vi "Update-references.vi"(6 "Control refs":refnum<vi>[](array[refnum]), 8 "error in (no error)":errorcluster, 9 "Sorted splitter references":refnum<vi>[](array[refnum]), 10 "Sorted pane references":refnum<vi>[](array[refnum]), 11 "Panes in":T1) -> (0 "error out":errorcluster, 3 "Panes out":T1)   [LabVIEW 2013, in "MaterialCharacterization.lvlib" / "MC-UI.lvclass"]
uses:
  MC-UI.lvclass
  Panes-reference.ctl
  MC-UI.lvclass/MC-UI.ctl
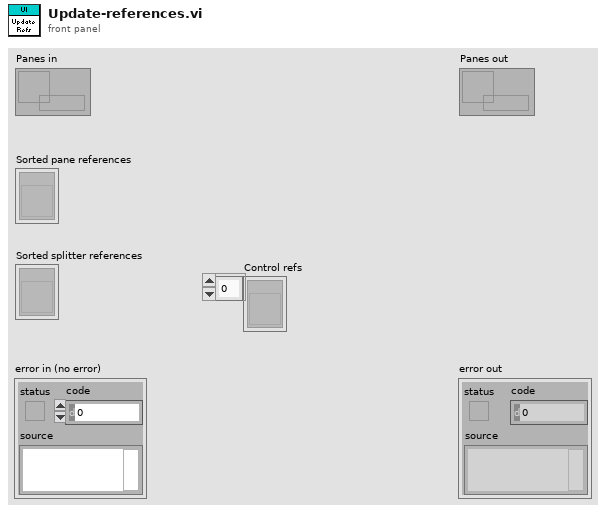
[diagram p1: front panel]
types:
  T1 = typedef "MaterialCharacterization.lvlib/MC-UI.lvclass/Panes-reference.ctl" = refnum<data-value>
  T2 = typedef "MaterialCharacterization.lvlib/HC-UI.lvclass/Pane-settings.ctl" = cluster{"Pane-name":T3, "Startup status":bool, "Current status":bool, "Splitters":T4[], "Pane-reference":refnum<vi>}
  T3 = typedef "MaterialCharacterization.lvlib/HC-UI.lvclass/Pane-names.ctl" = enum16{"Toolbar", "Help bar", "Toolbar lower border", "Center panel", "Main panel", "Settings panel", "Status bar upper border", "General state bar", "Information bar"}
  T4 = typedef "MaterialCharacterization.lvlib/HC-UI.lvclass/Splitter-settings.ctl" = cluster{"Splitter-name":T5, "Position shown":i32, "Position hidden":i32, "Splitter reference":refnum<vi>}
  T5 = typedef "MaterialCharacterization.lvlib/HC-UI.lvclass/Splitter-names.ctl" = enum16{"Upper toolbar splitter", "Help bar splitter", "Lower toolbar splitter", "Upper status bar splitter", "Lower status bar splitter", "Left status bar splitter", "Settings splitter"}
  T6 = typedef "MaterialCharacterization.lvlib/MC-UI.lvclass/Pane-settings.ctl" = cluster{"Pane-name":T7, "Startup status":bool, "Current status":bool, "Splitters":T8[], "Pane-reference":refnum<vi>}
  T7 = typedef "MaterialCharacterization.lvlib/MC-UI.lvclass/Pane-names.ctl" = enum16{"Toolbar", "Help bar", "Toolbar lower border", "Center panel", "Main panel", "Settings panel", "Status bar upper border", "General state bar", "Information bar"}
  T8 = typedef "MaterialCharacterization.lvlib/MC-UI.lvclass/Splitter-settings.ctl" = cluster{"Splitter-name":T9, "Position shown":i32, "Position hidden":i32, "Splitter reference":refnum<vi>}
  T9 = typedef "MaterialCharacterization.lvlib/MC-UI.lvclass/Splitter-names.ctl" = enum16{"Upper toolbar splitter", "Help bar splitter", "Lower toolbar splitter", "Upper status bar splitter", "Lower status bar splitter", "Left status bar splitter", "Settings splitter"}
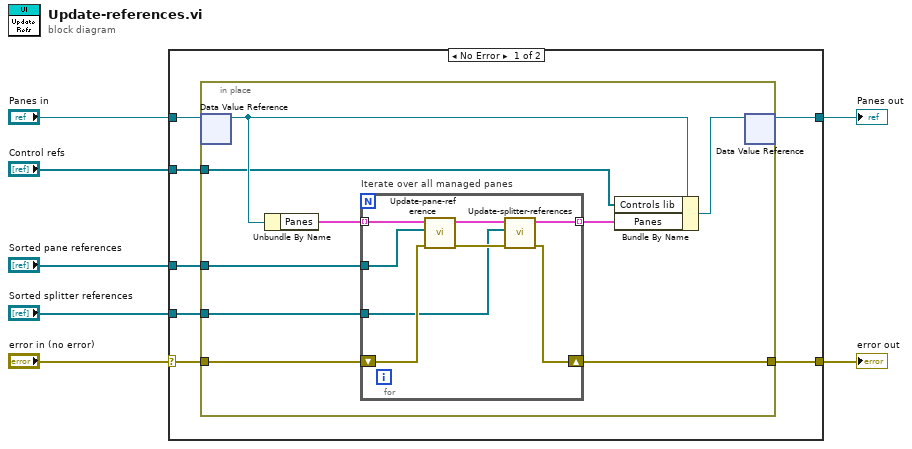
[diagram p0: block diagram]
diagram:
  n1 = case shown="No Error" "error in (no error)" {
    selector: "error in (no error)" -> [w13 w32]
    tunnel: [w12 w32] -> w6
    tunnel: [w9 w33] -> w4
    tunnel: "Panes in" -> [w10 w33]
    tunnel: "Sorted pane references" -> [w14 _]
    tunnel: "Sorted splitter references" -> [w11 _]
    tunnel: "Control refs" -> [w8 _]
    frame No Error {
      n2 = in-place {
        in-place-border: w14 -> [w23]
        in-place-border: w13 -> [w22]
        in-place-border: [w21] -> w12
        in-place-border: w11 -> [w20]
        in-place-border: w8 -> [w15]
        n3 = in-place-dvr #1(w10) -> (w17:refnum<class "MC-UI.lvclass">)  [unwired: 1 out]
        n4 = Unbundle By Name(w17) -> ("Panes"=w19:T2[])
        n5 = for "Iterate over all managed panes" {
          tunnel: w19 -> [w30] mode=indexing
          tunnel: w23 -> [w31]
          tunnel: w20 -> [w25]
          tunnel: [w27] -> w18 mode=indexing
          shift-right: [w24] -> w21
          shift-left: w22 -> [w29]
          n6 = call "Update-pane-reference.vi"("error in (no error)"=w29, "Sorted pane references"=w31, "Pane in"=w30) -> ("error out"=w26:errorcluster, "Pane out"=w28:T6)  [unwired: 7 in]
          n7 = call "Update-splitter-references.vi"("error in (no error)"=w26, "Sorted splitter references"=w25, "Pane in"=w28) -> ("error out"=w24:errorcluster, "Pane out"=w27:T6)  [unwired: 7 in]
        }
        n8 = Bundle By Name(cluster=w17, "Controls lib"=w15, "Panes"=w18) -> (w16:refnum<class "MC-UI.lvclass">)
        n9 = in-place-dvr #1(w16) -> (w9:T1)  [unwired: 1 out]
      }
    }
    frame Error {
    }
  }
  "error out" <- w6
  "Panes out" <- w4
